vi "Updata Current Mode.vi"(10 "Current Set Mode":string[][](array[string]), 11 "Current Set":u8[][](array[numeric])) -> (3 "Current Mode":u8[][](array[numeric]))   [LabVIEW 2023]
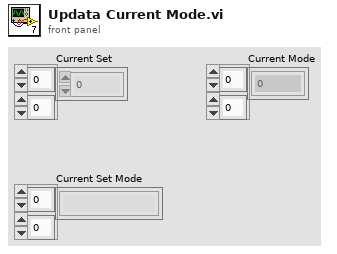
[diagram p1: front panel]
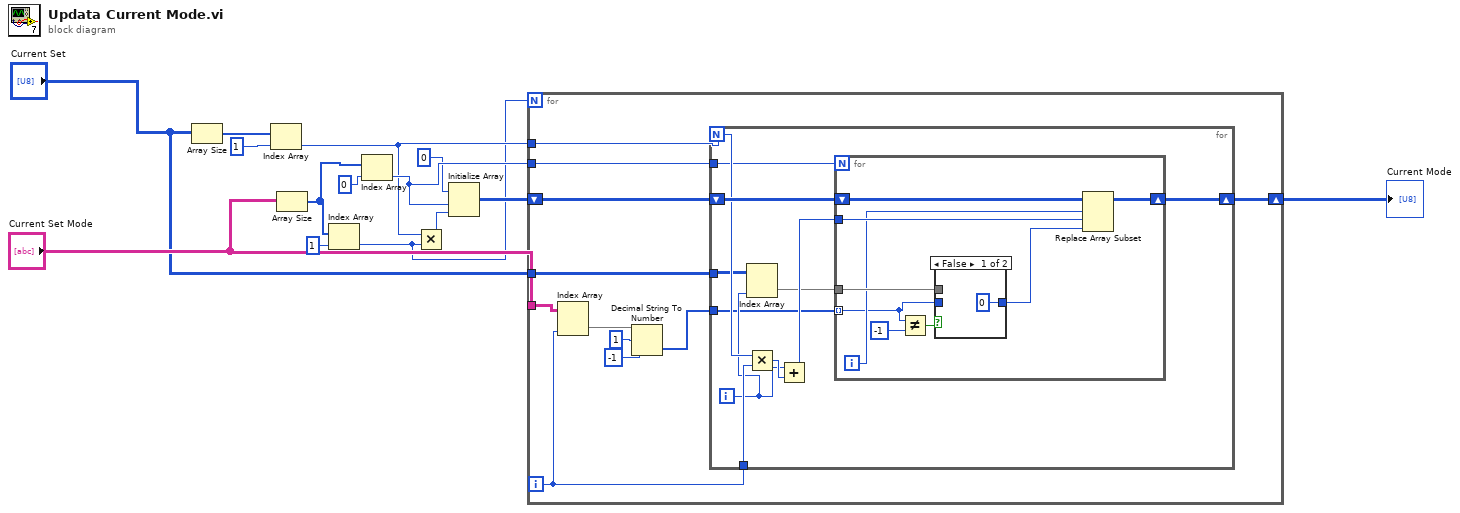
[diagram p0: block diagram]
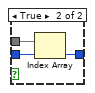
[diagram p2: hidden frame]
diagram:
  n1 = Array Size(array="Current Set") -> (size(s)=w1:i32[])
  n2 = Index Array(array=w1, index=1) -> (element=w9:i32)
  n3 = Array Size(array="Current Set Mode") -> (size(s)=w5:i32[])
  n4 = Index Array(array=w5, index=1) -> (element=w8:i32)
  n5 = Index Array(array=w5, index=0) -> (element=w12:i32)
  n6 = Multiply(x=w9, y=w8) -> (x*y=w6:i32)
  n7 = Initialize Array(u8 0 ("String"), w12, w6) -> (w10:u8[][])
  n8 = for {
    N: w8 -> [_]
    tunnel: w9 -> [w25]
    shift-right: [w22] -> w14
    shift-left: w10 -> [w23]
    tunnel: "Current Set" -> [w24]
    tunnel: w12 -> [w21]
    tunnel: "Current Set Mode" -> [w20]
    i -> [w19]
    n9 = Index Array(array=w20, index (col)=w19) -> (element=w17:string[])  [unwired: 1 in]
    n10 = Decimal String To Number(string=w17, offset=1, default (0L)=-1 ("default (0 I32)")) -> (number=w15:i32[])  [unwired: 1 out]
    n11 = for {
      N: w25 -> [w33]
      tunnel: w24 -> [w29]
      shift-right: [w31] -> w22
      shift-left: w23 -> [w36]
      tunnel: w19 -> [w34]
      tunnel: w21 -> [w30]
      tunnel: w15 -> [w26]
      i -> [w28]
      n12 = Index Array(array=w29, index (col)=w28) -> (element=w27:u8[])  [unwired: 1 in]
      n13 = Multiply(x=w33, y=w34) -> (x*y=w35:i32)
      n14 = Add(x=w28, y=w35) -> (x+y=w32:i32)
      n15 = for {
        N: w30 -> [_]
        tunnel: w32 -> [w44]
        shift-right: [w43] -> w31
        shift-left: w36 -> [w45]
        tunnel: w27 -> [w42]
        tunnel: w26 -> [w38] mode=indexing
        i -> [w41]
        n16 = Not Equal?(x=w38, y=-1) -> (x != y?=w39:bool)
        n17 = case shown="False" w39 {
          tunnel: w42 -> [_ w49]
          tunnel: w38 -> [_ w48]
          tunnel: [u8 0 ("String") w47] -> w40
          frame False {
          }
          frame True {
            n18 = Index Array(array=w49, index=w48) -> (element=w47:u8)
          }
        }
        n19 = Replace Array Subset(array=w45, new element=w40, index (row)=w41, index (col)=w44) -> (w43:u8[][])
      }
    }
  }
  "Current Mode" <- w14
